vi "TestExec.Add New 1D Items to 2D List, Overwrite if is existing.vi"(9 "New Items":string[][](array[string]), 11 "Item List":string[][](array[string])) -> (3 "Item List Out":string[][](array[string]))   [LabVIEW 2018]
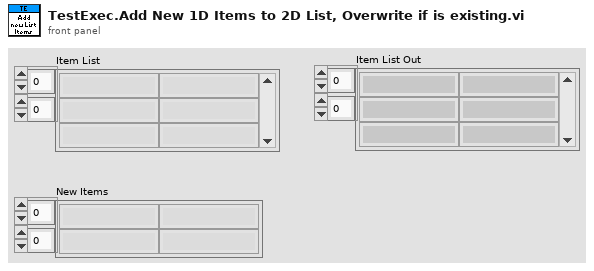
[diagram p1: front panel]
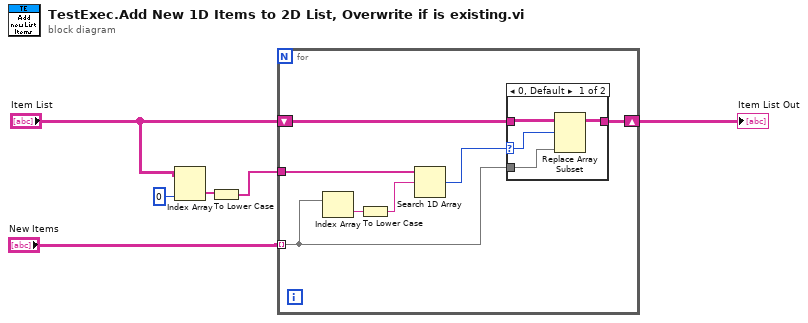
[diagram p0: block diagram]
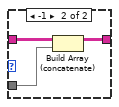
[diagram p2: hidden frame]
diagram:
  n1 = Index Array(array="Item List", index (col)=0 ("disabled index (col)")) -> (element=w2:string[])  [unwired: 1 in]
  n2 = To Lower Case(string=w2) -> (all lower case string=w1:string[])
  n3 = for {
    tunnel: "New Items" -> [w9] mode=indexing
    shift-right: [w12] -> w5
    shift-left: "Item List" -> [w13]
    tunnel: w1 -> [w10]
    n4 = Index Array(array=w9) -> (element=w8:string)  [unwired: 1 in]
    n5 = To Lower Case(string=w8) -> (all lower case string=w7:string)
    n6 = Search 1D Array(1D array=w10, element=w7) -> (index of element=w11:i32)  [unwired: 1 in]
    n7 = case shown="0, Default" w11 {
      selector: w11 -> [w14 _]
      tunnel: w13 -> [w17 w20]
      tunnel: [w16 w19] -> w12
      tunnel: w9 -> [w15 w18]
      frame 0, Default {
        n8 = Replace Array Subset(array=w17, new element=w15, index (row)=w14) -> (w16:string[][])  [unwired: 1 in]
      }
      frame -1 {
        n9 = Build Array (concatenate)(w20, w18) -> (w19:string[][])
      }
    }
  }
  "Item List Out" <- w5
